vi "create_spec_devices.vi"(8 "error in (no error)":errorcluster) -> (0 "error out":errorcluster)   [LabVIEW 2017]
doc: "reads settings for each MS in \"Massspectrometer.ini\" and creates objects for each of those devices. Those objects are stored in a global variable. The global variable stores any object no matter what type"
uses:
  Classes/Spectrometer/Spectrometer.lvclass
  global variables.vi
  <vilib>/Utility/config.llb/Read Key (String).vi
  Classes/StatusLog/StatusLog.lvclass
  <vilib>/Utility/config.llb/NI_LVConfig.lvlib
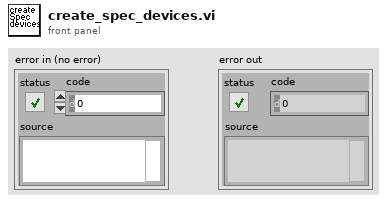
[diagram p1: front panel]
types:
  T1 = typedef "NI_LVConfig.lvlib/Config Data RefNum.ctl" = refnum<k1>
  T2 = typedef "Semaphore RefNum" = refnum<k1>
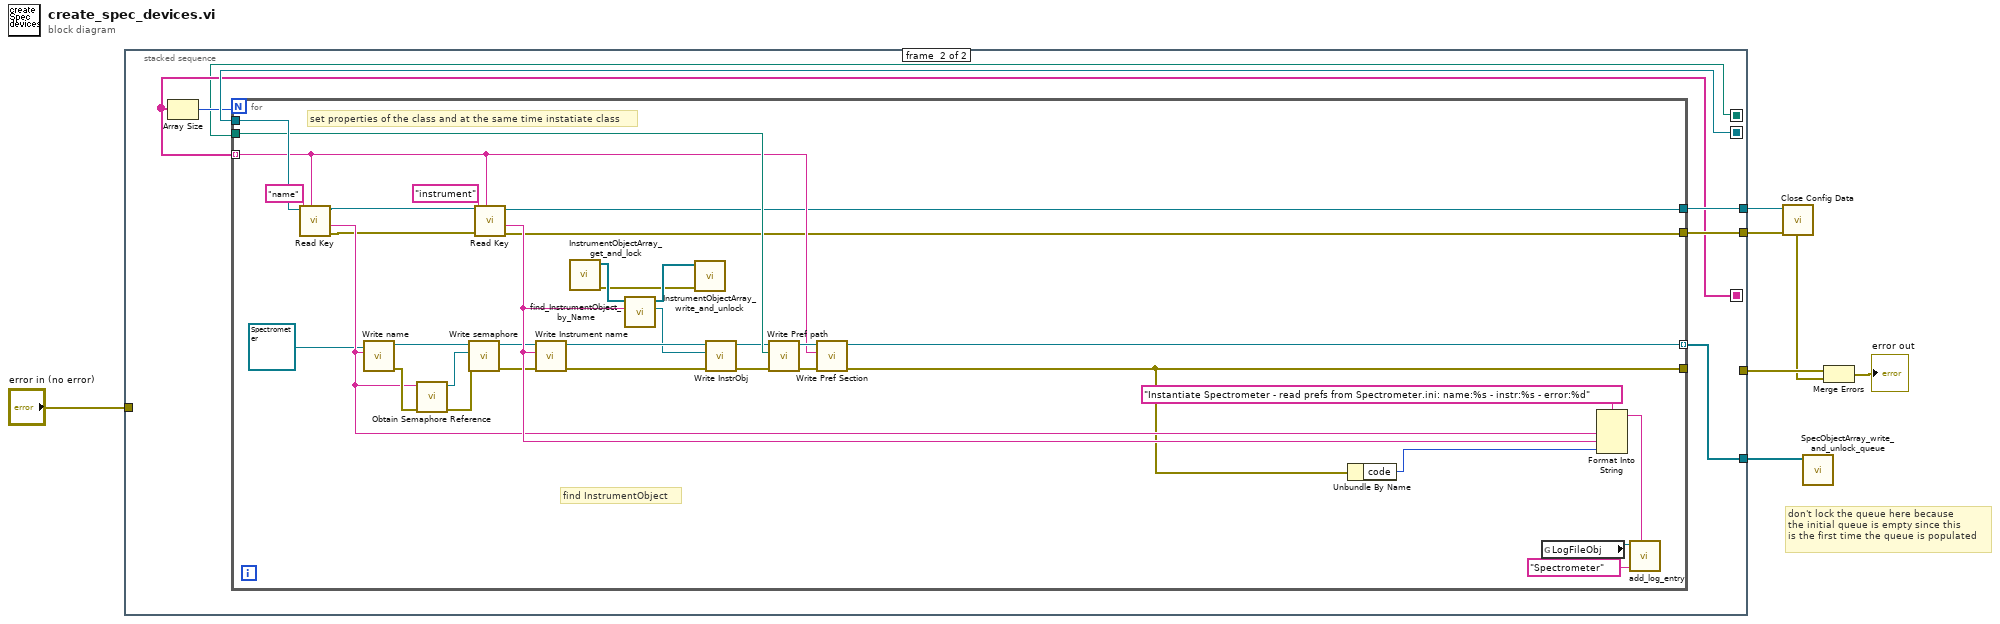
[diagram p0: block diagram]
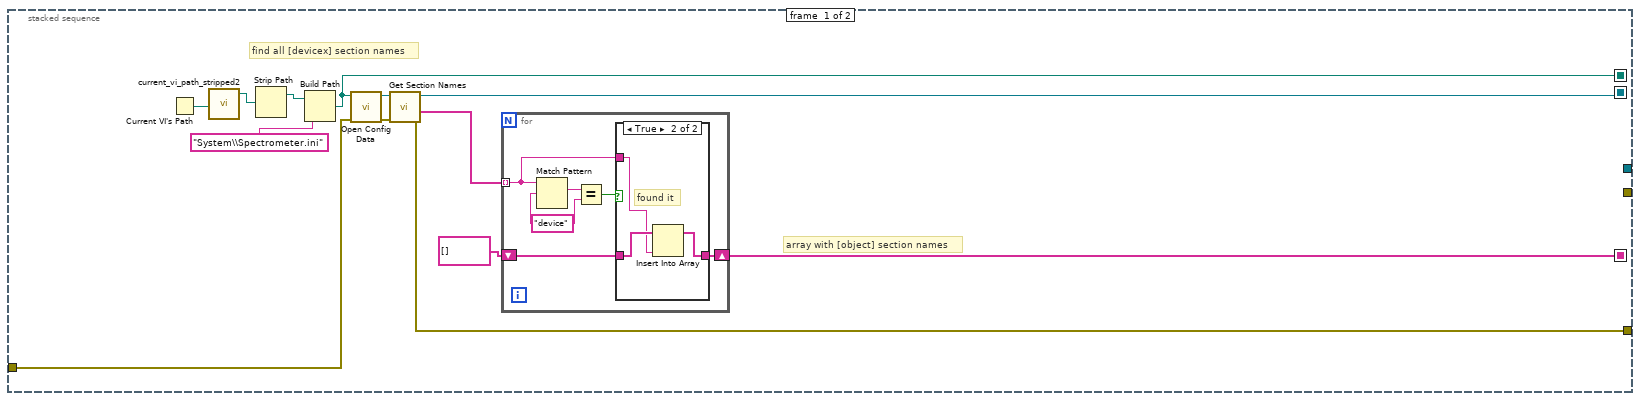
[diagram p2: hidden frame]
diagram:
  # "don't lock the queue here because\nthe initial queue is empty since this\nis the first time the queue is populated"
  n1 = stacked-sequence {
    seq-local: [w16 _] -> [_ w37]
    seq-local: [w12 _] -> [_ w33]
    seq-local: [w11 _] -> [_ w32]
    tunnel: "error in (no error)" -> [w17 _]
    tunnel: [w15 _] -> w6
    tunnel: [_ w36] -> w4
    tunnel: [_ w35] -> w3
    tunnel: [_ w31] -> w1
    frame #0 {
      # "array with [object] section names"
      # "find all [devicex] section names"
      n2 = Current VI's Path() -> (path=w10:path)
      n3 = call "current_vi_path_stripped2.vi"("current VI Path"=w10) -> ("current VI Path stripped out"=w8:path)  [unwired: 3 in, 1 out]
      n4 = Strip Path(path=w8) -> (stripped path=w9:path)  [unwired: 1 out]
      n5 = Build Path(base path=w9, name or relative path="System\\Spectrometer.ini") -> (appended path=w11:path)
      n6 = call <vilib>:"Open Config Data.vi"("error in (no error)"=w17, "configuration file path"=w11) -> ("error out"=w18:errorcluster, "refnum"=w19:T1)  [unwired: 7 in, 1 out]
      n7 = call <vilib>:"Get Section Names.vi"("error in (no error)"=w18, "refnum"=w19) -> ("error out"=w15:errorcluster, "section names"=w14:string[], "refnum out"=w16:T1)  [unwired: 7 in]
      n8 = for {
        tunnel: w14 -> [w23] mode=indexing
        shift-right: [w21] -> w12
        shift-left: string[] [] ("section names") -> [w22]
        w25 = "device" ("regular expression")
        n9 = Match Pattern(string=w23, regular expression=w25) -> (match substring=w26:string)  [unwired: 1 in, 3 out]
        n10 = Equal?(x=w26, y=w25) -> (x = y?=w24:bool)
        n11 = case shown="True" w24 {
          tunnel: w23 -> [_ w29]
          tunnel: [w27 w28] -> w21
          tunnel: w22 -> [w27 w30]
          frame False {
            # "no match"
          }
          frame True {
            # "found it"
            n12 = Insert Into Array(array=w30, new element=w29) -> (w28:string[])  [unwired: 1 in]
          }
        }
      }
    }
    frame #1 {
      n13 = Array Size(array=w33) -> (size(s)=w34:i32)
      n14 = for {
        N: w34 -> [_]
        tunnel: w37 -> [w72]
        tunnel: [w52] -> w36
        tunnel: [w51] -> w35
        tunnel: w33 -> [w53] mode=indexing
        tunnel: w32 -> [w67]
        tunnel: [w45] -> w31 mode=indexing
        tunnel: [w43] -> _
        # "find InstrumentObject"
        # "set properties of the class and at the same time instatiate class"
        n15 = call-poly <vilib>:"Read Key.vi"("section"=w53, "key"="name", "refnum"=w72) -> ("error out"=w46:errorcluster, "value"=w55:string, "refnum out"=w47:T1)  [unwired: 5 in, 1 out]
        n16 = call-dynamic "Write name.vi"("name"=w55, "Spectrometer in"=refnum<class "Spectrometer.lvclass"> refnum ("Spectrometer.lvclass")) -> ("error out"=w57:errorcluster, "Spectrometer out"=w58:refnum<class "Spectrometer.lvclass">)  [unwired: 8 in]
        n17 = call <vilib>:"Obtain Semaphore Reference.vi"("error in (no error)"=w57, "name (unnamed)"=w55) -> ("error out"=w56:errorcluster, "semaphore"=w54:T2)  [unwired: 3 in, 1 out]
        n18 = call-dynamic "Write semaphore.vi"("error in (no error)"=w56, "semaphore"=w54, "Spectrometer in"=w58) -> ("error out"=w48:errorcluster, "Spectrometer out"=w49:refnum<class "Spectrometer.lvclass">)  [unwired: 7 in]
        n19 = call-poly <vilib>:"Read Key.vi"("section"=w53, "error in (no error)"=w46, "key"="instrument", "refnum"=w47) -> ("error out"=w51:errorcluster, "value"=w59:string, "refnum out"=w52:T1)  [unwired: 4 in, 1 out]
        n20 = call-dynamic "Write Instrument name.vi"("error in (no error)"=w48, "Instrument name"=w59, "Spectrometer in"=w49) -> ("error out"=w62:errorcluster, "Spectrometer out"=w63:refnum<class "Spectrometer.lvclass">)  [unwired: 7 in]
        n21 = call "InstrumentObjectArray_get_and_lock.vi"() -> ("error out"=w38:errorcluster, "InstrumentsObjects"=w40:refnum<class "instrument.lvclass">[])  [unwired: 10 in]
        n22 = call "find_InstrumentObject_by_Name.vi"("Instrument Name"=w59, "InstrumentObjects"=w40) -> ("found InstrObject out"=w41:refnum<class "instrument.lvclass">, "InstrumentObjects out"=w39:refnum<class "instrument.lvclass">[])  [unwired: 6 in, 2 out]
        n23 = call "InstrumentObjectArray_write_and_unlock.vi"("error in (no error)"=w38, "InstrumentObjects"=w39) -> ()  [unwired: 9 in, 1 out]
        n24 = call-dynamic "Write InstrObj.vi"("error in (no error)"=w62, "instrument.lvclass"=w41, "Spectrometer in"=w63) -> ("error out"=w60:errorcluster, "Spectrometer out"=w61:refnum<class "Spectrometer.lvclass">)  [unwired: 7 in]
        n25 = call-dynamic "Write Pref path.vi"("error in (no error)"=w60, "Pref path"=w67, "Spectrometer in"=w61) -> ("error out"=w68:errorcluster, "Spectrometer out"=w69:refnum<class "Spectrometer.lvclass">)  [unwired: 7 in]
        n26 = call-dynamic "Write Pref Section.vi"("error in (no error)"=w68, "Pref Section"=w53, "Spectrometer in"=w69) -> ("error out"=w43:errorcluster, "Spectrometer out"=w45:refnum<class "Spectrometer.lvclass">)  [unwired: 7 in]
        n27 = Unbundle By Name(w43) -> ("code"=w42:i32)
        n28 = global read "global variables.vi" "LogFileObj"() -> (w66:refnum<class "StatusLog.lvclass">)
        n29 = Format Into String(format string="Instantiate Spectrometer - read prefs from Spectrometer.ini: name:%s - instr:%s - error:%d", w55, w59, w42) -> (resulting string=w64:string)  [unwired: 2 in, 1 out]
        n30 = call-dynamic "add_log_entry.vi"("new entry"=w64, "log identifiers"="Spectrometer", "StatusLog in"=w66) -> ()  [unwired: 5 in, 2 out]
      }
    }
  }
  n31 = call <vilib>:"Close Config Data.vi"("error in (no error)"=w3, "refnum"=w4) -> ("error out"=w2:errorcluster)  [unwired: 8 in, 1 out]
  n32 = call "SpecObjectArray_write_and_unlock_queue.vi"("PrepLineObjArray"=w1) -> ()  [unwired: 10 in, 1 out]
  n33 = Merge Errors(w6, w2) -> (→"error out":errorcluster)
